vi "Run_5_of_X_Tests.vi"() -> ()   [LabVIEW 2019]
uses:
  <vilib>/Rock Robotics/WPI/ThirdParty/JAS_Junk/TrajLib/Trajectory_Library.lvlib
panel:
  out "String":string
  out "All Tests Finished":bool
  out "Diff Drive Train Sim":bool
  out "DARE - Ricatti":bool
  out "Discretization":bool
  # "FORMAL TRAJECTORY / CONTROL LIBRARY TEST PROCEDURE"
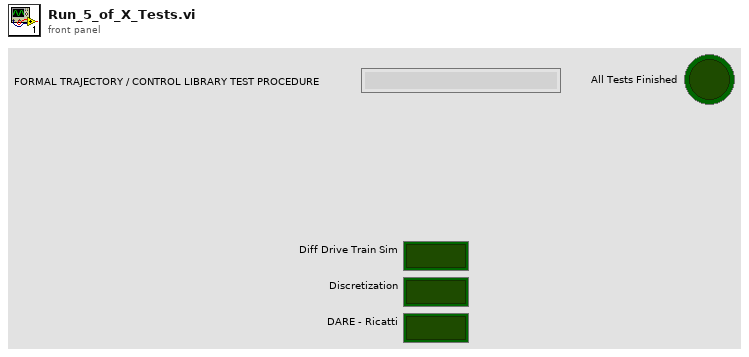
[diagram p1: front panel]
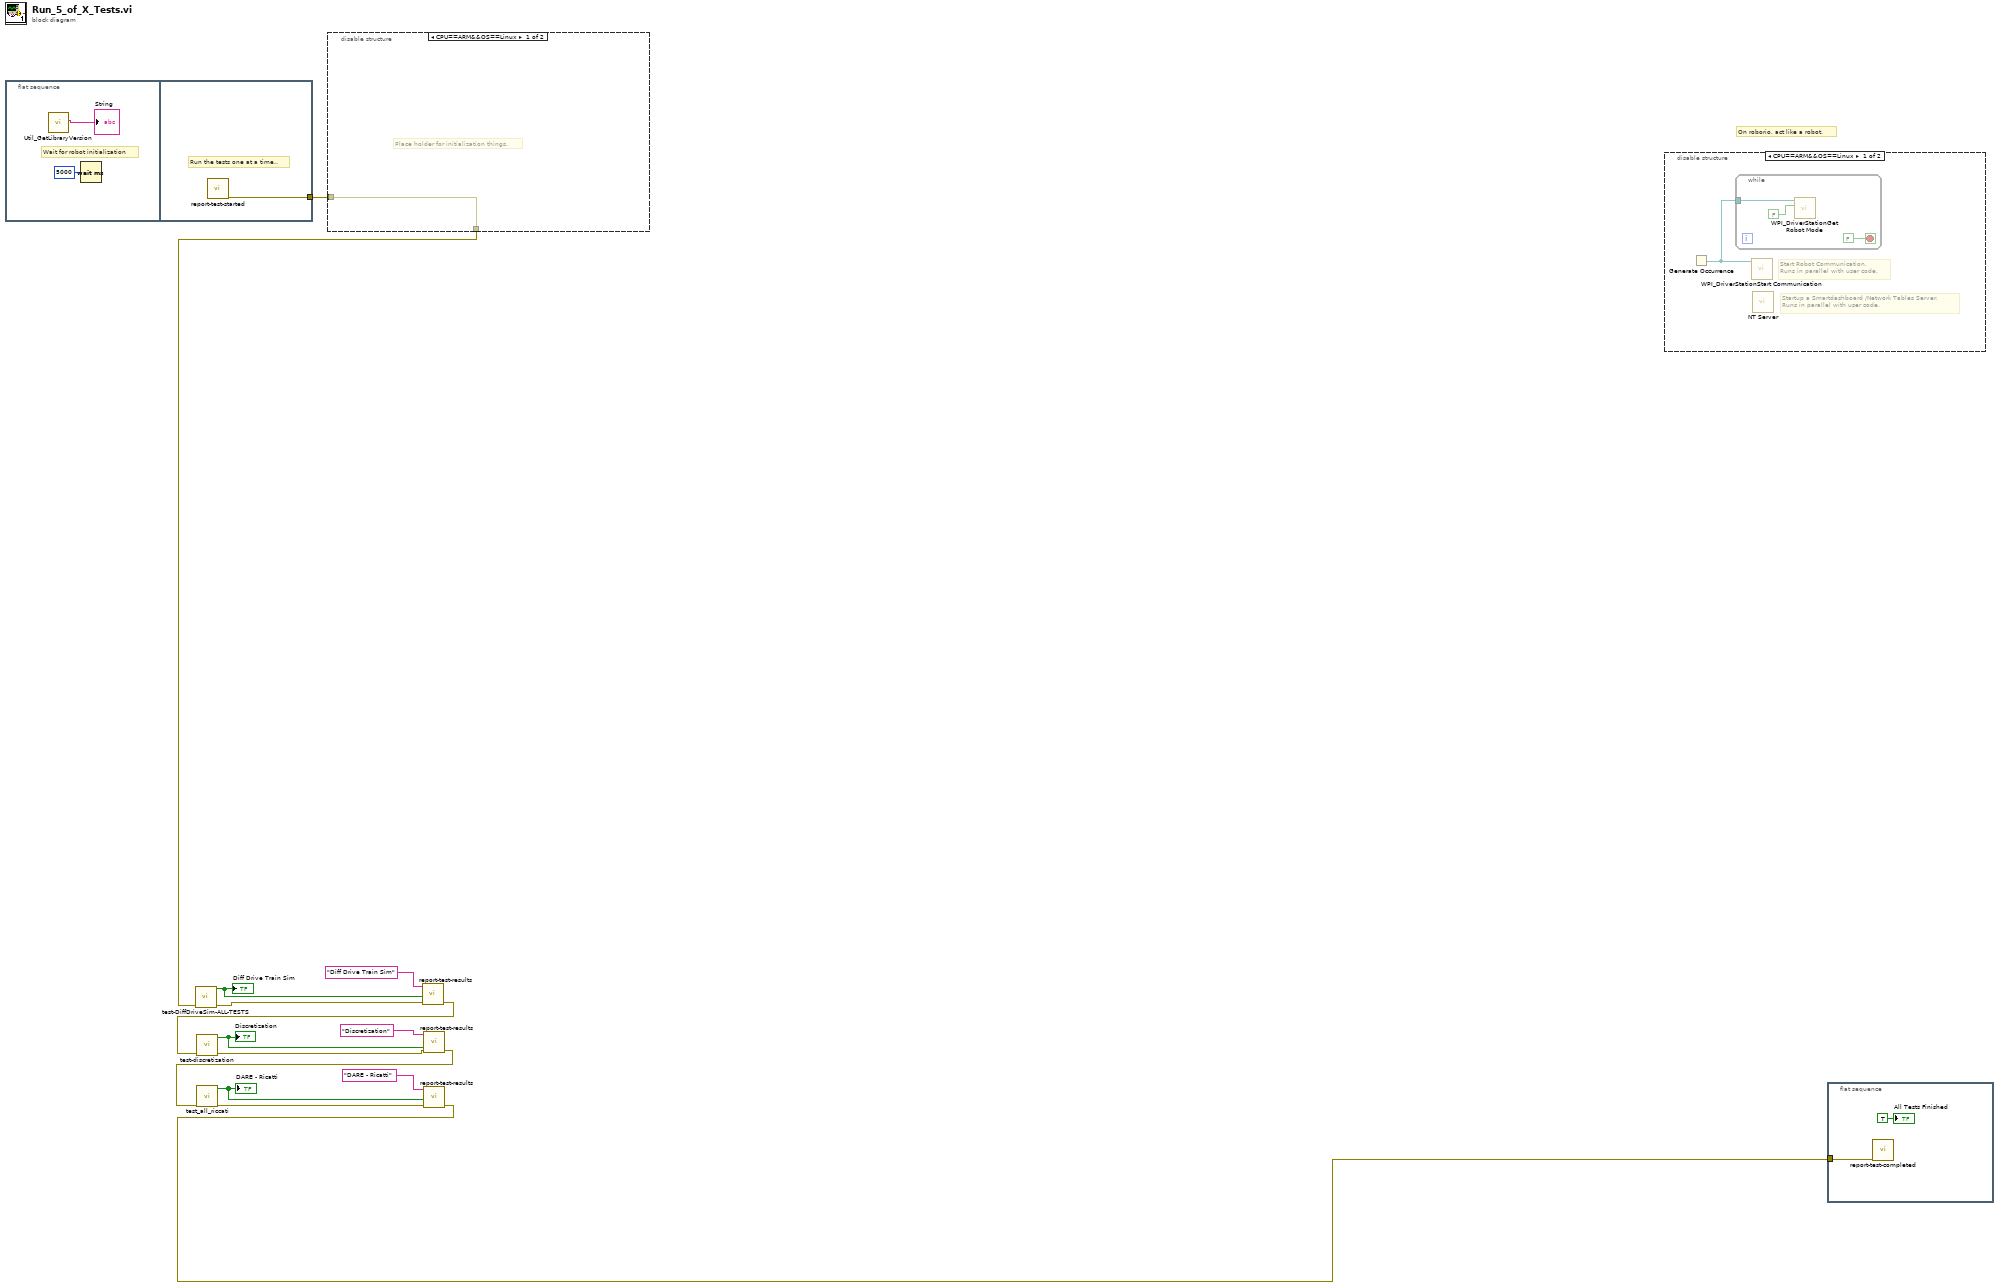
[diagram p0: block diagram]
diagram:
  # "On roborio, act like a robot."
  n1 = flat-sequence {
    tunnel: [w17] -> w3
    frame #0 {
      # "Wait for robot initialization"
      n2 = call <vilib>:"Util_GetLibraryVersion.vi"() -> ("TrajLibVersion"=→"String":string)  [unwired: 11 in]
      n3 = Wait (ms)(milliseconds to wait=u32 5000) -> ()  [unwired: 1 out]
    }
    frame #1 {
      # "Run the tests one at a time.."
      n4 = call "report-test-started.vi"() -> ("error out"=w17:errorcluster)  [unwired: 11 in]
    }
  }
  n5 = disable-structure shown="CPU==ARM&&OS==Linux" {
    disable-tunnel: w3 -> [w18 w19]
    disable-tunnel: [w18 w19] -> w2
    frame condition #0 {
      # "Place holder for initialization things."
    }
    frame condition #1 (active) {
    }
  }
  n6 = call "test-DiffDriveSim-ALL-TESTS.vi"("error in (no error)"=w2) -> ("error out"=w6:errorcluster, "All Passed"=w11:bool)  [unwired: 9 in]
  "Diff Drive Train Sim" <- w11
  n7 = call "report-test-results.vi"("error in (no error)"=w6, "TestPassed"=w11, "Test Name"="Diff Drive Train Sim") -> ("error out"=w4:errorcluster)  [unwired: 8 in]
  n8 = call "test-discretization.vi"("error in (no error)"=w4) -> ("error out"=w8:errorcluster, "All Tests Passed"=w10:bool)  [unwired: 9 in]
  "Discretization" <- w10
  n9 = call "report-test-results.vi"("error in (no error)"=w8, "TestPassed"=w10, "Test Name"="Discretization") -> ("error out"=w7:errorcluster)  [unwired: 8 in]
  n10 = call "test_all_riccati.vi"("error in (no error)"=w7) -> ("error out"=w5:errorcluster, "All Tests Passed"=w9:bool)  [unwired: 9 in]
  "DARE - Ricatti" <- w9
  n11 = call "report-test-results.vi"("error in (no error)"=w5, "TestPassed"=w9, "Test Name"="DARE - Ricatti") -> ("error out"=w1:errorcluster)  [unwired: 8 in]
  n12 = disable-structure shown="CPU==ARM&&OS==Linux" {
    frame condition #0 {
      # "Startup a Smartdashboard /Network Tables Server.\nRuns in parallel with user code."
      # "Start Robot Communication.\nRuns in parallel with user code."
      n13 = Generate Occurrence() -> (w20:refnum<k4>)
      n14 = while {
        tunnel: w20 -> [w23]
        stop <- FALSE stop-if-true
        n15 = call <vilib>:"WPI_DriverStationGet Robot Mode.vi"("Finish"=FALSE, "DS Occurrence"=w23) -> ()  [unwired: 10 out]
      }
      n16 = call <vilib>:"WPI_DriverStationStart Communication.vi"("occurrence"=w20) -> ()  [unwired: 2 in, 9 out]
      n17 = call <vilib>:"NT Server.vi"() -> ()  [unwired: 12 in]
    }
    frame condition #1 (active) {
    }
  }
  n18 = flat-sequence {
    tunnel: w1 -> [w24]
    frame #0 {
      n19 = call "report-test-completed.vi"("error in (no error)"=w24) -> ()  [unwired: 10 in, 1 out]
      "All Tests Finished" <- TRUE ("All Tests Finished")
    }
  }
